vi "LCA Get Dev Err Msg.vi"(8 "error in (no error)":errorcluster caption="Fehler (Eingang, kein Fehler)", 10 "Error Code":i32, 11 "Axis Handle":i64) -> (0 "error out":errorcluster caption="Fehler (Ausgang)", 3 "Error Message":string)   [LabVIEW 2021, in "labbCAN_MotionControl_API.lvlib"]
doc: "LCA_Func long __stdcall LCA_GetDevErrMsg(dev_hdl hAxis,\n long DevErr,\n char *pStringBuf,\n short BufSize);"
uses:
  labbCAN_MotionControl_API.lvlib
  labbCAN_MotionControl_API.dll
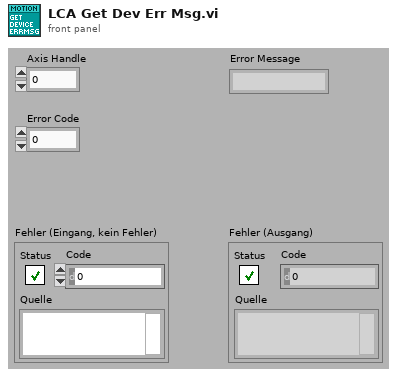
[diagram p1: front panel]
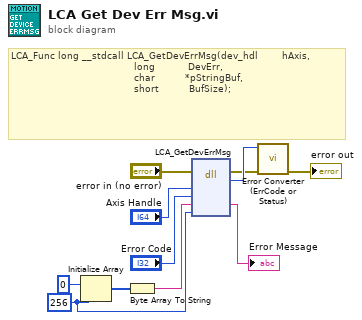
[diagram p0: block diagram]
diagram:
  w1 = 256 ("Dimension")
  # "LCA_Func long __stdcall LCA_GetDevErrMsg(dev_hdl        hAxis,\n                                         long           DevErr,\n                                         char          *pStringBuf,\n                                         short          BufSize);"
  n1 = Initialize Array(u8 0 ("Element"), w1) -> (w8:u8[])
  n2 = Byte Array To String(unsigned byte array=w8) -> (string=w7:string)
  n3 = dll-call lib="C:/Users/olaja/AppData/Local/CETONI_SDK/labbCAN_MotionControl_API.*" fn="LCA_GetDevErrMsg"(error in="error in (no error)", "hAxis"="Axis Handle", "DevErr"="Error Code", "pStringBuf"=w7, "BufSize"=w1) -> (error out=w3:errorcluster, "Rückgabetyp"=w11:i32, "pStringBuf"=→"Error Message":string)  [unwired: 5 in, 1 out]
  n4 = call "Error Converter (ErrCode or Status).vi"("error in (no error)"=w3, "error code"=w11) -> ("error out"=→"error out":errorcluster)  [unwired: 9 in]
